vi "replase property.vi"() -> ()   [LabVIEW 2019]
panel:
  in  "name":string
  out "Array":errorcluster[](array[cluster])
  out "subarray":string[](array[string])
  out "array":string[][](array[string])
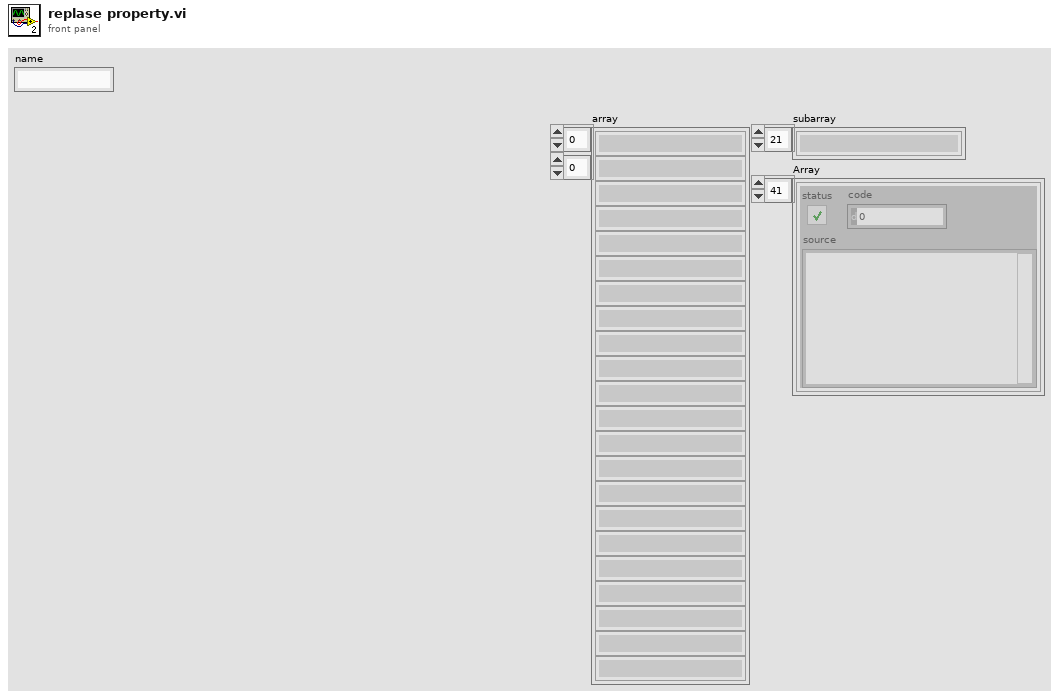
[diagram p1: front panel]
types:
  T1 = enum16{"Share clones between instances", "Preallocate clone for each instance"}
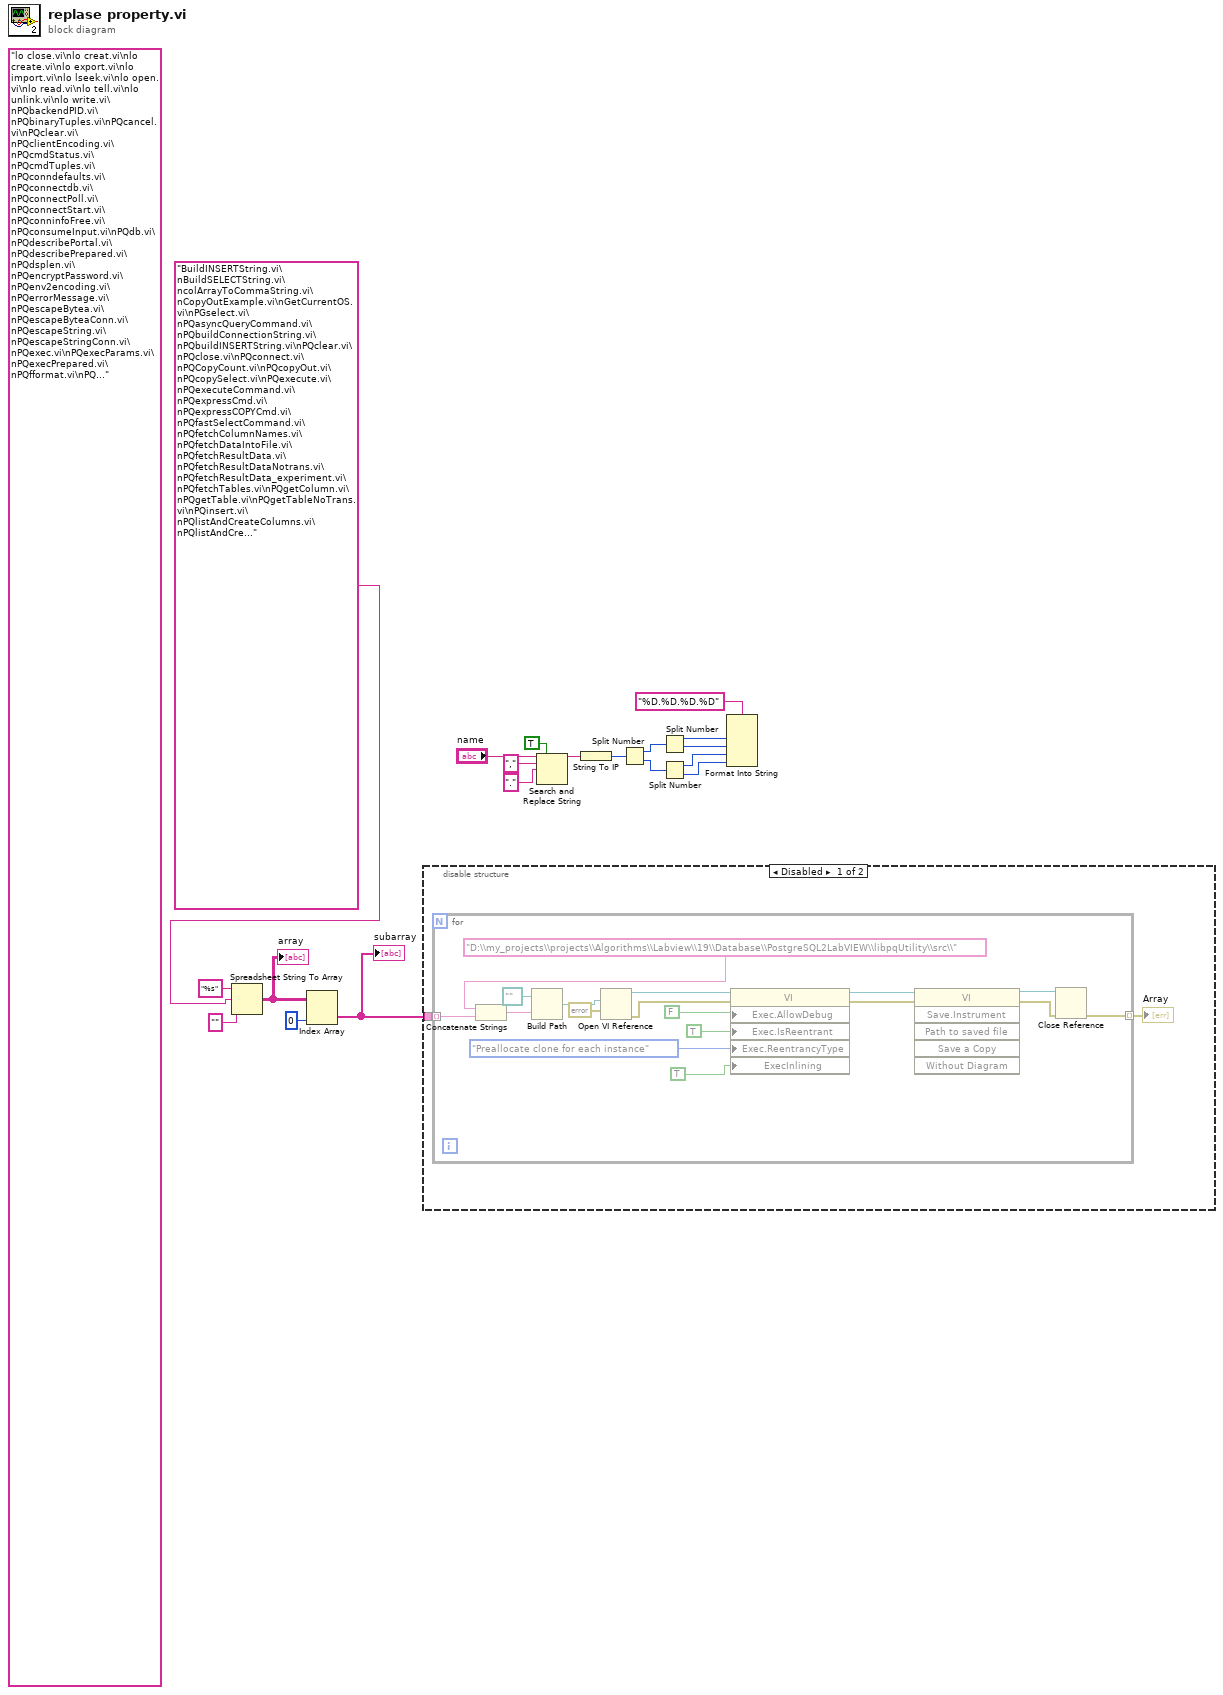
[diagram p0: block diagram]
diagram:
  (unwired) "lo close.vi\nlo creat.vi\nlo create.vi\nlo export.vi\nlo import.vi\nlo lseek.vi\nlo open.vi\nlo read.vi\nlo tell.vi\nlo unlink.vi\nlo write.vi\nPQbackendPID.vi\nPQbinaryTuples.vi\nPQcancel.vi\nPQclear.vi\nPQclientEncoding.vi\nPQcmdStatus.vi\nPQcmdTuples.vi\nPQconndefaults.vi\nPQconnectdb.vi\nPQconnectPoll.vi\nPQconnectStart.vi\nPQconninfoFree.vi\nPQconsumeInput.vi\nPQdb.vi\nPQdescribePortal.vi\nPQdescribePrepared.vi\nPQdsplen.vi\nPQencryptPassword.vi\nPQenv2encoding.vi\nPQerrorMessage.vi\nPQescapeBytea.vi\nPQescapeByteaConn.vi\nPQescapeString.vi\nPQescapeStringConn.vi\nPQexec.vi\nPQexecParams.vi\nPQexecPrepared.vi\nPQfformat.vi\nPQfinish.vi\nPQflush.vi\nPQfmod.vi\nPQfname.vi\nPQfnumber.vi\nPQfreeCancel.vi\nPQfreemem.vi\nPQfsize.vi\nPQftable.vi\nPQftablecol.vi\nPQftype.vi\nPQgetCancel.vi\nPQgetCopyData.vi\nPQgetisnull.vi\nPQgetlength.vi\nPQgetResult.vi\nPQgetssl.vi\nPQgetvalue.vi\nPQhost.vi\nPQinitSSL.vi\nPQisBusy.vi\nPQisnonblocking.vi\nPQisthreadsafe.vi\nPQmakeEmptyPGresult.vi\nPQmblen.vi\nPQnfields.vi\nPQnotifies.vi\nPQnparams.vi\nPQntuples.vi\nPQoidStatus.vi\nPQoidValue.vi\nPQoptions.vi\nPQparameterStatus.vi\nPQparamtype.vi\nPQpass.vi\nPQport.vi\nPQprepare.vi\nPQprint.vi\nPQprotocolVersion.vi\nPQputCopyData.vi\nPQputCopyEnd.vi\nPQregisterThreadLock.vi\nPQrequestCancel.vi\nPQreset.vi\nPQresetPoll.vi\nPQresetStart.vi\nPQresStatus.vi\nPQresultErrorField.vi\nPQresultErrorMessage.vi\nPQresultStatus.vi\nPQsendDescribePortal.vi\nPQsendDescribePrepared.vi\nPQsendPrepare.vi\nPQsendQuery.vi\nPQsendQueryParams.vi\nPQsendQueryPrepared.vi\nPQserverVersion.vi\nPQsetClientEncoding.vi\nPQsetdbLogin.vi\nPQsetErrorVerbosity.vi\nPQsetnonblocking.vi\nPQsetNoticeProcessor.vi\nPQsetNoticeReceiver.vi\nPQsocket.vi\nPQstatus.vi\nPQtransaction Status.vi\nPQtty.vi\nPQunescapeBytea.vi\nPQuntrace.vi\nPQuser.vi"
  n1 = Spreadsheet String To Array(format string="%s", spreadsheet string="BuildINSERTString.vi\nBuildSELECTString.vi\ncolArrayToCommaString.vi\nCopyOutExample.vi\nGetCurrentOS.vi\nPGselect.vi\nPQasyncQueryCommand.vi\nPQbuildConnectionString.vi\nPQbuildINSERTString.vi\nPQclear.vi\nPQclose.vi\nPQconnect.vi\nPQCopyCount.vi\nPQcopyOut.vi\nPQcopySelect.vi\nPQexecute.vi\nPQexecuteCommand.vi\nPQexpressCmd.vi\nPQexpressCOPYCmd.vi\nPQfastSelectCommand.vi\nPQfetchColumnNames.vi\nPQfetchDataIntoFile.vi\nPQfetchResultData.vi\nPQfetchResultDataNotrans.vi\nPQfetchResultData_experiment.vi\nPQfetchTables.vi\nPQgetColumn.vi\nPQgetTable.vi\nPQgetTableNoTrans.vi\nPQinsert.vi\nPQlistAndCreateColumns.vi\nPQlistAndCreateSequence.vi\nPQlistColumns.vi\nPQlistSequenses.vi\nPQlistTables.vi\nPQopen.vi\nPQselect.vi\nPQselect_Sample.vi\nPQsetClientEncoding.vi\nPQsyncQueryCommand.vi\nPQ_asynchron_sample.vi\nPQ_synchron_sample.vi\nValidateSELECTInputs.vi", array type (2D Dbl)="" ("format string")) -> (array=w17:string[][])  [unwired: 1 in]
  "array" <- w17
  n2 = Index Array(array=w17, index (col)=0 ("index (row)")) -> (element=w15:string[])  [unwired: 1 in]
  "subarray" <- w15
  n3 = disable-structure shown="Disabled" {
    disable-tunnel: w15 -> [w21 _]
    frame Disabled {
      n4 = for {
        tunnel: w21 -> [w24] mode=indexing
        tunnel: [w23] -> w20 mode=indexing
        n5 = Concatenate Strings("D:\\my_projects\\projects\\Algorithms\\Labview\\19\\Database\\PostgreSQL2LabVIEW\\libpqUtility\\src\\", w24) -> (w26:string)
        n6 = Build Path(base path=path "", name or relative path=w26) -> (appended path=w25:path)
        n7 = Open VI Reference(vi path=w25, error in (no error)=errorcluster {"status"=FALSE, "code"=0, "source"=""}) -> (vi reference=w38:refnum<vi>, error out=w37:errorcluster)  [unwired: 4 in]
        n8 = property class="VI"(reference=w38, error in=w37, "Exec.AllowDebug"=FALSE ("Execution:Allow Debugging"), "Exec.IsReentrant"=TRUE ("Execution:Is Reentrant"), "Exec.ReentrancyType"=T1."Preallocate clone for each instance" ("Execution:Reentrancy Type"), "ExecInlining"=TRUE ("Execution:Is Reentrant")) -> (reference out=w32:refnum<vi>, error out=w29:errorcluster)
        n9 = invoke class="VI" method="Save.Instrument"(reference=w32, error in=w29) -> (reference out=w31:refnum<vi>, error out=w30:errorcluster)  [unwired: 4 in, 4 out]
        n10 = Close Reference(reference=w31, error in (no error)=w30) -> (error out=w23:errorcluster)
      }
      "Array" <- w20
    }
    frame Enabled {
    }
  }
  n11 = Search and Replace String(replace all?=TRUE ("replace all? (F)"), input string="name", search string=",", replace string="." ("replace string (\"\")")) -> (result string=w2:string)  [unwired: 4 in, 3 out]
  n12 = String To IP(1:w2) -> (0:w13:u32)
  n13 = Split Number(x=w13) -> (hi(x)=w12:u16, lo(x)=w11:u16)
  n14 = Split Number(x=w12) -> (hi(x)=w9:u8, lo(x)=w8:u8)
  n15 = Split Number(x=w11) -> (hi(x)=w7:u8, lo(x)=w6:u8)
  n16 = Format Into String(format string="%D.%D.%D.%D", w9, w8, w7, w6) -> ()  [unwired: 2 in, 2 out]
